vi "Set Servo Angle.vi"(8 "error in (no error)":errorcluster, 9 "Angle (0 - 180)":sgl, 10 "GPIO":i32, 11 "VISA resource name in":refnum<visa-resource-name>) -> (0 "error out":errorcluster, 3 "VISA resource name":refnum<visa-resource-name>)   [LabVIEW 2023, in "CTI-Visa.lvlib"]
uses:
  CTI-Visa.lvlib
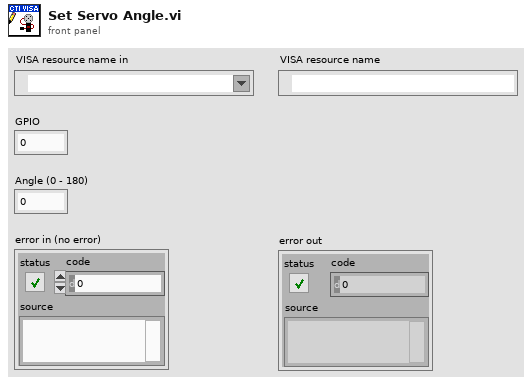
[diagram p1: front panel]
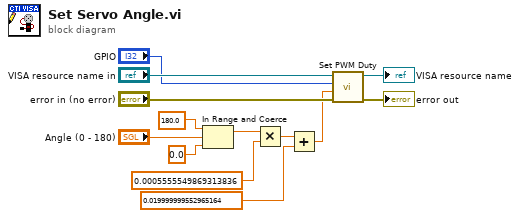
[diagram p0: block diagram]
diagram:
  n1 = In Range and Coerce(upper limit=sgl 180.0, x="Angle (0 - 180)", lower limit=sgl 0.0) -> (coerced(x)=w10:sgl)  [unwired: 1 out]
  n2 = Multiply(x=w10, y=sgl 0.000555555) -> (x*y=w8:sgl)
  n3 = Add(x=w8, y=sgl 0.02) -> (x+y=w3:sgl)
  n4 = call "Set PWM Duty.vi"("error in (no error)"="error in (no error)", "Duty % (0-1)"=w3, "Channel"="GPIO", "VISA resource name in"="VISA resource name in") -> ("error out"=→"error out":errorcluster, "VISA resource name"=→"VISA resource name":refnum<visa-resource-name>)  [unwired: 6 in]
